vi "Digital IO polymorphe 2.vi"() -> ()   [LabVIEW 2020]
uses:
  <userlib>/DAQNavi Polymorphic VI/create/DAQNavi Create Channel(DO-Digital Output).vi
  <userlib>/DAQNavi Polymorphic VI/create/DAQNavi Create Channel(DI-Digital Input).vi
  <userlib>/DAQNavi Polymorphic VI/write/DAQNavi Write (Digital U8 1Chan 1Samp).vi
  <userlib>/DAQNavi Polymorphic VI/read/DAQNavi Read (Digital U8 1Chan 1Samp).vi
panel:
  out "DI":u8
  out "DO":u8
  in  "Stop":bool
  in  "DO":u8
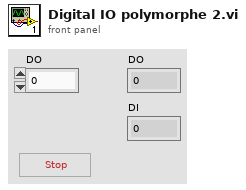
[diagram p1: front panel]
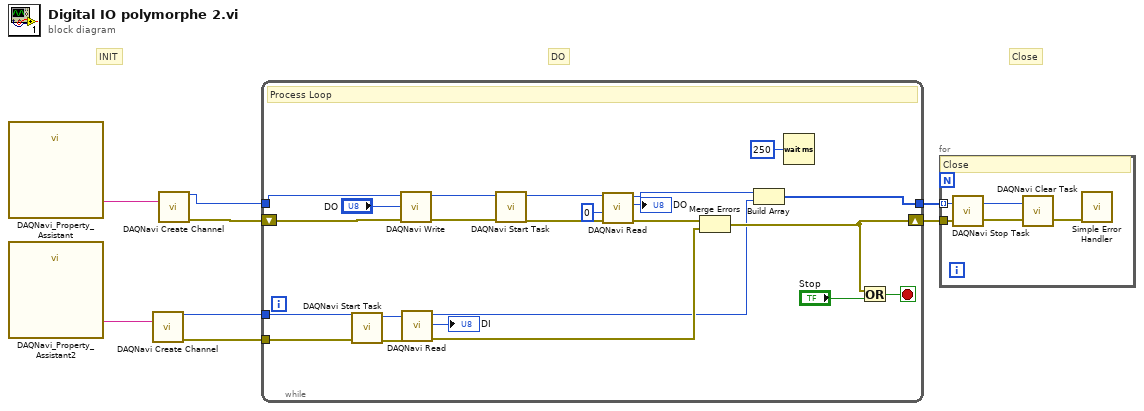
[diagram p0: block diagram]
diagram:
  # "Close"
  # "DO"
  # "INIT"
  n1 = call "DAQNavi_Property_Assistant"() -> ("property value"=w8:string)  [unwired: 1 in]
  n2 = call "DAQNavi_Property_Assistant2"() -> ("property value"=w1:string)  [unwired: 1 in]
  n3 = call-poly <userlib>:"DAQNavi Create Channel.vi"("physical channels"=w1) -> ("task out"=w2:i32, "error out"=w3:errorcluster)  [unwired: 13 in]
  n4 = call-poly <userlib>:"DAQNavi Create Channel.vi"("physical channels"=w8) -> ("task out"=w5:i32, "error out"=w4:errorcluster)  [unwired: 13 in]
  n5 = while {
    shift-right: [w13] -> w7
    shift-left: w4 -> [w24]
    tunnel: w3 -> [w18]
    tunnel: w2 -> [w16]
    tunnel: w5 -> [w25]
    tunnel: [w11] -> w6
    stop <- w20 stop-if-true
    # "Process Loop"
    n6 = call <userlib>:"DAQNavi Start Task.vi"("error in (no error)"=w18, "task in"=w16) -> ("error out"=w17:errorcluster, "task out"=w15:i32)  [unwired: 8 in]
    n7 = call-poly <userlib>:"DAQNavi Write.vi"("error in (no error)"=w24, "data"="DO", "task in"=w25) -> ("error out"=w26:errorcluster, "task out"=w27:i32)  [unwired: 6 in, 1 out]
    n8 = call-poly <userlib>:"DAQNavi Read.vi"("error in (no error)"=w17, "task in"=w15) -> ("error out"=w12:errorcluster, "data"=→"DI":u8, "task out"=w10:i32)  [unwired: 7 in]
    n9 = call <userlib>:"DAQNavi Start Task.vi"("error in (no error)"=w26, "task in"=w27) -> ("error out"=w30:errorcluster, "task out"=w31:i32)  [unwired: 8 in]
    n10 = call-poly <userlib>:"DAQNavi Read.vi"("error in (no error)"=w30, "portBit"=0, "task in"=w31) -> ("error out"=w22:errorcluster, "data"=→"DO":u8, "task out"=w29:i32)  [unwired: 6 in]
    n11 = Merge Errors(w22, w12) -> (w13:errorcluster)
    n12 = Build Array(w29, w10) -> (w11:i32[])
    n13 = Wait (ms)(milliseconds to wait=u32 250) -> ()  [unwired: 1 out]
    n14 = Or(x=w13, y="Stop") -> (x .or. y?=w20:bool)
  }
  n15 = for {
    tunnel: w7 -> [w34]
    tunnel: w6 -> [w33] mode=indexing
    # "Close"
    n16 = call <userlib>:"DAQNavi Stop Task.vi"("error in (no error)"=w34, "task in"=w33) -> ("error out"=w35:errorcluster, "task out"=w36:i32)
    n17 = call <userlib>:"DAQNavi Clear Task.vi"("error in (no error)"=w35, "task in"=w36) -> ("error out"=w32:errorcluster)  [unwired: 1 in]
    n18 = call <vilib>:"Simple Error Handler.vi"("error in (no error)"=w32) -> ()  [unwired: 4 in, 5 out]
  }
